vi "Add Recent Project.vi"(8 "error in (no error)":errorcluster, 10 "New Recent Experiment path":path, 11 "User Preferences File in":refnum<class "User Preferences File.lvclass">) -> (0 "error out":errorcluster, 3 "User Preferences File out":refnum<class "User Preferences File.lvclass">)   [LabVIEW 2020, in "User Preferences File.lvclass"]
doc: "Adds a new path to the Recent Experiments list. This Recent Experiment list is kept in chronological order, so the newly added Recent Experiment will always be at the top. If the new experiment already exists, the old entry is removed and the new entry is placed at the top of the Recent Experiments list."
uses:
  User Preferences File.lvclass
  User Preferences File.lvclass/User Preferences File.ctl
  8a9409e5-1c3d-4ac7-bb6e-67f5d1127aba.vi
  <vilib>/Comparison/Equal/Equal Functor/Equal Functor.lvclass
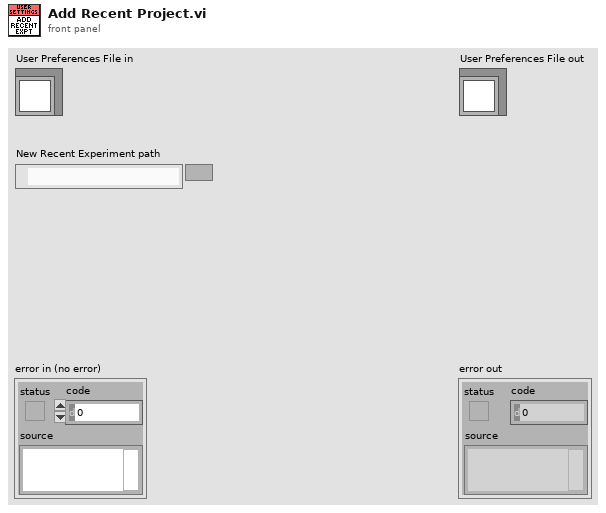
[diagram p1: front panel]
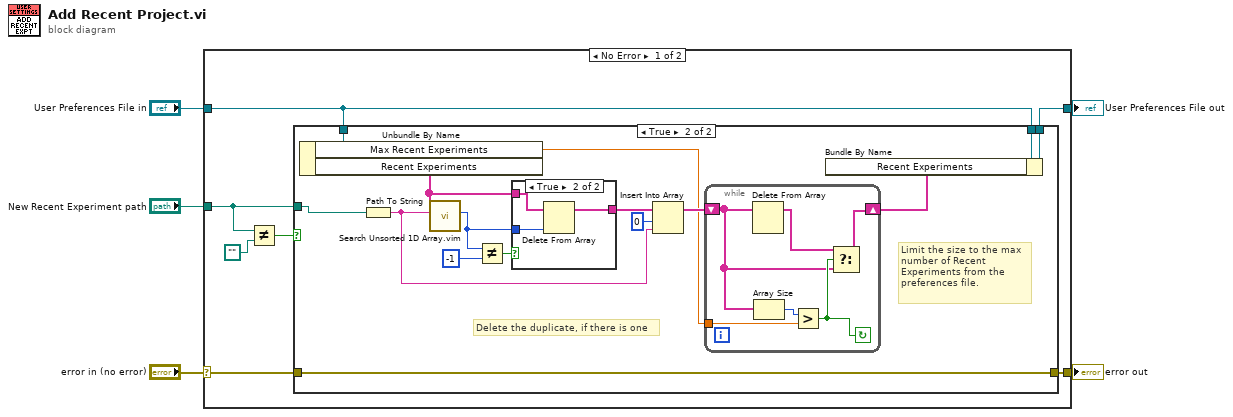
[diagram p0: block diagram]
diagram:
  n1 = case shown="No Error" "error in (no error)" {
    selector: "error in (no error)" -> [w11 w41]
    tunnel: [w6 w41] -> w4
    tunnel: [w7 w40] -> w2
    tunnel: "User Preferences File in" -> [w8 w40]
    tunnel: "New Recent Experiment path" -> [w9 _]
    frame No Error {
      n2 = Not Equal?(x=w9, y=path "") -> (x != y?=w10:bool)
      n3 = case shown="True" w10 {
        tunnel: w8 -> [_ w29]
        tunnel: w11 -> [w13 w18]
        tunnel: w9 -> [_ w28]
        tunnel: w8 -> [w14 w20]
        tunnel: [w14 w19] -> w7
        tunnel: [w13 w18] -> w6
        frame False {
        }
        frame True {
          # "Limit the size to the max\nnumber of Recent\nExperiments from the \npreferences file."
          # "Delete the duplicate, if there is one"
          n4 = Unbundle By Name(w29) -> ("Max Recent Experiments"=w16:dbl, "Recent Experiments"=w27:string[])
          n5 = Path To String(path=w28) -> (string=w21:string)
          n6 = call "Search Unsorted 1D Array.vim"("element"=w21, "unsorted 1D array"=w27) -> ("index of element"=w24:i32)  [unwired: 9 in]
          n7 = Not Equal?(x=w24, y=-1) -> (x != y?=w26:bool)
          n8 = case shown="True" w26 {
            tunnel: w24 -> [_ w39]
            tunnel: w27 -> [w36 w38]
            tunnel: [w36 w37] -> w23
            frame False {
            }
            frame True {
              n9 = Delete From Array(array=w38, index=w39) -> (array with subset deleted=w37:string[])  [unwired: 1 in, 1 out]
            }
          }
          n10 = Insert Into Array(array=w23, index=0, new element=w21) -> (w17:string[])
          n11 = while {
            tunnel: w16 -> [w34]
            shift-right: [w30] -> w15
            shift-left: w17 -> [w32]
            stop <- w33 continue-if-true
            n12 = Delete From Array(array=w32) -> (array with subset deleted=w31:string[])  [unwired: 2 in, 1 out]
            n13 = Array Size(array=w32) -> (size(s)=w35:i32)
            n14 = Greater?(x=w35, y=w34) -> (0:w33:bool)
            n15 = Select(t=w31, s=w33, f=w32) -> (s? t:f=w30:string[])
          }
          n16 = Bundle By Name(cluster=w20, "Recent Experiments"=w15) -> (w19:refnum<class "User Preferences File.lvclass">)
        }
      }
    }
    frame Error {
    }
  }
  "error out" <- w4
  "User Preferences File out" <- w2
